vi "merFISH_initialize_Z_ramp_FPGA.vi"(0 "queue DAQ":refnum<queue>, 1 "queue piezo":refnum<queue>, 2 "queue CAMERA":refnum<queue>, 5 "Variant data":T3, 7 "Data cluster":T1, 11 "error in":errorcluster) -> (3 "Ramp":dbl[](array[numeric]), 4 "PATH cluster":T2, 15 "error out":errorcluster)   [LabVIEW 2015]
uses:
  CONTROLS/Q_DAQ_element.ctl
  CONTROLS/Q_MCL_piezo_element.ctl
  CONTROLS/Q_camera_element.ctl
  GLOBAL/Global_MAIN.vi
  GLOBAL/Global_MCL_piezo.vi
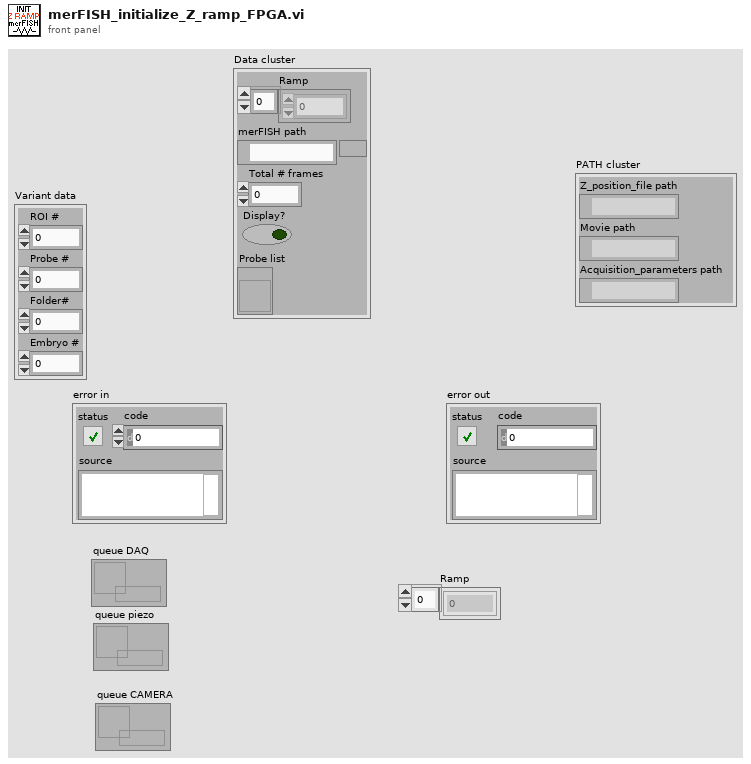
[diagram p1: front panel]
types:
  T1 = cluster{"Ramp":dbl[], "merFISH path":path, "Total # frames":i32, "Display?":bool, "Probe list":refnum<vi>}
  T2 = cluster{"Z_position_file path":path, "Movie path":path, "Acquisition_parameters path":path}
  T3 = cluster{"ROI #":i32, "Probe #":i32, "Folder# ":i32, "Embryo #":i32}
  T4 = cluster{"Movie path":path, "Total # frames":i32, "Display?":bool}
  T5 = typedef "Q_camera_element.ctl" = cluster{"variant":variant, "Instruction":enum16{"CAMERA_idle", "CAMERA_initialize", "CAMERA_error", "CAMERA_security_stop", "CAMERA_not_acquiring", "CAMERA_acquiring", "CAMERA_start_acquiring", "CAMERA_stop_acquiring", "CAMERA_change_exposure", "CAMERA_define_ROI", "CAMERA_cooler", "CAMERA_acquire_movie", "CAMERA_init_scan", "CAMERA_check_image_scan", "CAMERA_close_scan", "CAMERA_init_merFISH", "CAMERA_start_acquiring_merFISH", "CAMERA_close_scan_merFISH", "CAMERA_close_merFISH", "CAMERA_STOP"}}
  T6 = typedef "Q_MCL_piezo_element.ctl" = cluster{"variant":variant, "Instruction":enum16{"Piezo_idle", "Piezo_initialize", "Piezo_error", "Piezo_security_stop", "Piezo_read_z", "Piezo_move_z", "Piezo_keyboard_move", "Piezo_close_autofocus_calibration_ramp", "Piezo_change_init_state", "Piezo_init_autofocus", "Piezo_init_autofocus_merFISH_TL", "Piezo_autofocus", "Piezo_autofocus_merFISH_TL", "Piezo_stop_autofocus", "Piezo_stop_autofocus_merFISH_TL", "Piezo_autofocus_lost", "Piezo_resume_autofocus_merFISH_TL", "Piezo_check_z_position_merFISH_TL", "Piezo_init_ramp", "Piezo_move_z_ramp", "Piezo_close_ramp", "Piezo_close_merFISH", "Piezo_stop"}}
  T7 = typedef "Q_DAQ_element.ctl" = cluster{"variant":variant, "Instruction":enum16{"DAQ_idle", "DAQ_initialize", "DAQ_error", "DAQ_security_stop", "DAQ_init_single_scan", "DAQ_single_scan", "DAQ_init_merFISH", "DAQ_scan_merFISH", "DAQ_photobleaching_merFISH", "DAQ_close_merFISH", "DAQ_stop"}}
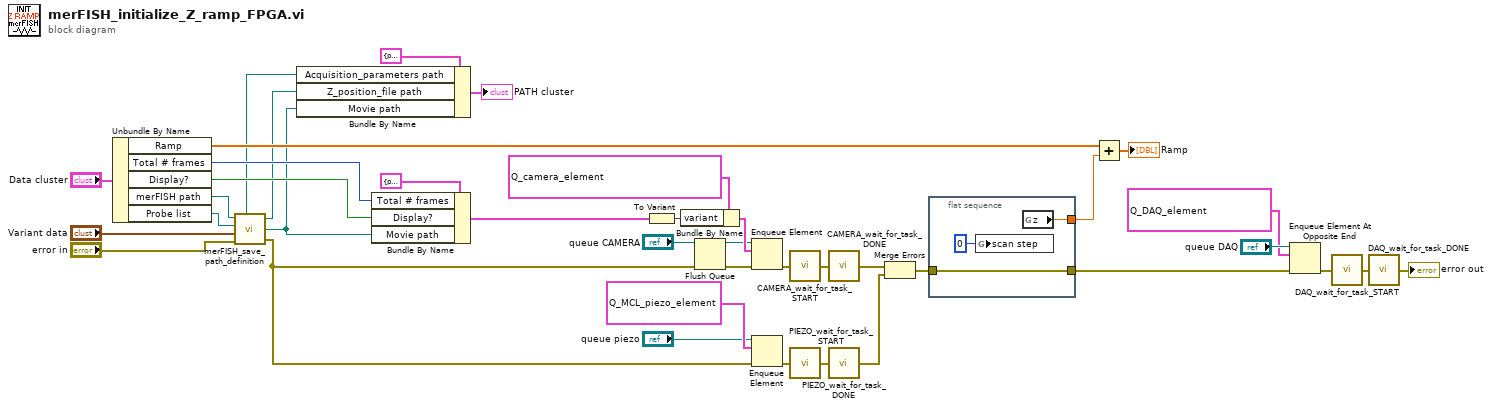
[diagram p0: block diagram]
diagram:
  n1 = Unbundle By Name("Data cluster") -> ("Ramp"=w33:dbl[], "Total # frames"=w15:i32, "Display?"=w16:bool, "merFISH path"=w17:path, "Probe list"=w3:refnum<vi>)
  n2 = call "merFISH_save_path_definition.vi"("merFISH path"=w17, "List probe Refnum"=w3, "Data"="Variant data", "error in"="error in") -> ("Acquisition_parameters path"=w11:path, "Z_position_file path"=w10:path, "Movie path"=w9:path, "error out"=w13:errorcluster)
  n3 = Bundle By Name(cluster=T2 {"Z_position_file path"=path "", "Movie path"=path "", "Acquisition_parameters path"=path ""} ("output cluster"), "Acquisition_parameters path"=w11, "Z_position_file path"=w10, "Movie path"=w9) -> (→"PATH cluster":T2)
  n4 = Bundle By Name(cluster=T4 {"Movie path"=path "", "Total # frames"=0, "Display?"=FALSE} ("output cluster"), "Total # frames"=w15, "Display?"=w16, "Movie path"=w9) -> (w18:T4)
  n5 = To Variant(anything=w18) -> (Variant=w26:variant)
  n6 = Bundle By Name(cluster=T5 {"variant"=variant, "Instruction"=enum."CAMERA_start_acquiring_merFISH"} ("Q_ANDOR_element"), "variant"=w26) -> (w27:T5)
  n7 = Flush Queue(queue="queue CAMERA", error in (no error)=w13) -> (queue out=w23:refnum<queue>, error out=w22:errorcluster)  [unwired: 1 out]
  n8 = Enqueue Element(queue=w23, element=w27, error in (no error)=w22) -> (error out=w24:errorcluster)  [unwired: 1 in, 2 out]
  n9 = Enqueue Element(queue="queue piezo", element=T6 {"variant"=variant, "Instruction"=enum."Piezo_init_ramp"}, error in (no error)=w13) -> (error out=w32:errorcluster)  [unwired: 1 in, 2 out]
  n10 = call "CAMERA_wait_for_task_START.vi"("error in"=w24) -> ("error out"=w25:errorcluster)
  n11 = call "PIEZO_wait_for_task_START.vi"("error in"=w32) -> ("error out"=w31:errorcluster)
  n12 = call "CAMERA_wait_for_task_DONE.vi"("error in"=w25) -> ("error out"=w7:errorcluster)
  n13 = call "PIEZO_wait_for_task_DONE.vi"("error in"=w31) -> ("error out"=w6:errorcluster)
  n14 = Merge Errors(w7, w6) -> (w5:errorcluster)
  n15 = flat-sequence {
    tunnel: w5 -> [w42]
    tunnel: [w42] -> w2
    tunnel: [w41] -> w1
    frame #0 {
      n16 = global write "Global_MAIN.vi" "scan step"(0 ("scan step")) -> ()
      n17 = global read "Global_MCL_piezo.vi" "z"() -> (w41:dbl)
    }
  }
  n18 = Add(x=w33, y=w1) -> (x+y=→"Ramp":dbl[])
  n19 = Enqueue Element At Opposite End(queue="queue DAQ", element=T7 {"variant"=variant, "Instruction"=enum."DAQ_init_single_scan"}, error in (no error)=w2) -> (error out=w36:errorcluster)  [unwired: 1 in, 2 out]
  n20 = call "DAQ_wait_for_task_START.vi"("error in"=w36) -> ("error out"=w37:errorcluster)
  n21 = call "DAQ_wait_for_task_DONE.vi"("error in"=w37) -> ("error out"=→"error out":errorcluster)
